vi "GetSimulatedYaw.vi"(4 "Real IMU Yaw (deg)":dbl format="%#_13g", 5 "Rotation Command":dbl, 6 "Auto Test Mode":bool, 7 "Max Simulated Rotation Speed (deg/s)":dbl, 8 "Reset Yaw (deg)":dbl format="%#_13g", 11 "Reset Yaw":bool) -> (1 "Simulated Yaw (deg)":dbl)   [LabVIEW 2019]
doc: "This VI simulates an IMU yaw reading based on the current drive base rotation command. It is intended for use when when testing autonomous plays on the robot cart. Pose pushes and resets are handled identically to the real IMU yaw sensor."
uses:
  <vilib>/Rock Robotics/WPI/DriverStation/WPI_DriverStationRobotMode2.ctl
  dsdata.vi
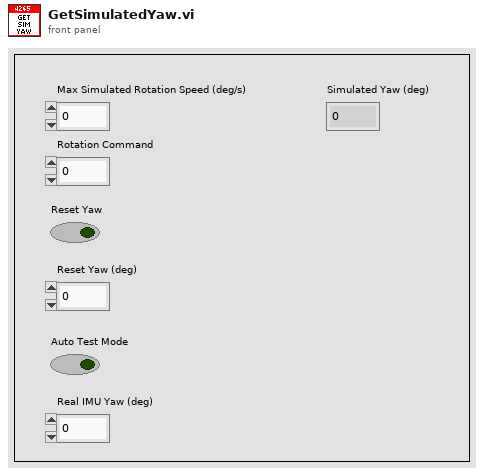
[diagram p1: front panel]
types:
  T1 = typedef "WPI_DriverStationRobotMode2.ctl" = enum16{"Autonomous Disabled", "Autonomous Enabled", "Teleop Disabled", "Teleop Enabled", "Disconnected", "Finish", "Test Disabled", "Test Enabled", "Emergency Stopped"}
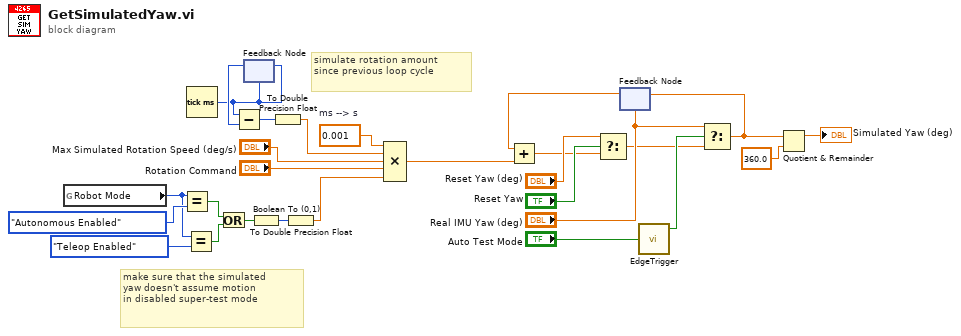
[diagram p0: block diagram]
diagram:
  w18 = 0.001  # ms --> s
  # "make sure that the simulated\nyaw doesn't assume motion\nin disabled super-test mode"
  # "simulate rotation amount\nsince previous loop cycle"
  n1 = global read "dsdata.vi" "Robot Mode"() -> (w7:T1)
  n2 = Equal?(x=w7, y=WPI_DriverStationRobotMode2."Autonomous Enabled") -> (x = y?=w4:bool)
  n3 = Equal?(x=w7, y=WPI_DriverStationRobotMode2."Teleop Enabled") -> (x = y?=w5:bool)
  n4 = Tick Count (ms)() -> (millisecond timer value=w14:u32)
  n5 = Or(x=w4, y=w5) -> (x .or. y?=w3:bool)
  n6 = feedback #1(w14) -> (w15:u32)
  n7 = Subtract(x=w14, y=w15) -> (x-y=w16:u32)
  n8 = feedback-in #1(w14) -> ()
  n9 = Boolean To (0,1)(Boolean=w3) -> (0, 1=w2:i16)
  n10 = To Double Precision Float(number=w16) -> (double precision float=w17:dbl)
  n11 = To Double Precision Float(number=w2) -> (double precision float=w1:dbl)
  n12 = Compound Arithmetic op=MULTIPLY(w18, w17, "Max Simulated Rotation Speed (deg/s)", "Rotation Command", w1) -> (w11:dbl)
  n13 = feedback #2("Real IMU Yaw (deg)") -> (w10:dbl)
  n14 = Add(x=w10, y=w11) -> (x+y=w19:dbl)
  n15 = Select(t="Reset Yaw (deg)", s="Reset Yaw", f=w19) -> (s? t:f=w20:dbl)
  n16 = call "EdgeTrigger.vi"("Input Signal"="Auto Test Mode") -> ("Rising Edge Trigger"=w25:bool)  [unwired: 2 out]
  n17 = Select(t="Real IMU Yaw (deg)", s=w25, f=w20) -> (s? t:f=w21:dbl)
  n18 = feedback-in #2(w21) -> ()
  n19 = Quotient & Remainder(x=w21, y=360.0) -> (x-y*floor(x/y)=→"Simulated Yaw (deg)":dbl)  [unwired: 1 out]
